vi "LOG Initialize Hardware References.vi"(8 "error in (no error)":errorcluster, 10 "Message Data":variant, 11 "Hardware Resources in":T1) -> (0 "error out":errorcluster, 3 "Hardware Resources out":T1)   [LabVIEW 2020, in "LOG.lvlib"]
doc: "Initialize the hardware references."
uses:
  LOG.lvlib
  LOG Configuration.ctl
  support/Message Queue/Message Cluster.ctl
  support/Message Queue/Message Queue.lvlib
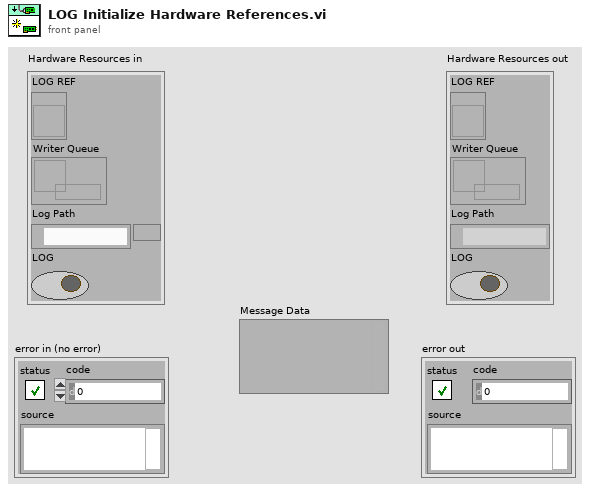
[diagram p1: front panel]
types:
  T1 = typedef "LOG.lvlib/LOG Configuration.ctl" = cluster{"LOG REF":refnum<vi>, "Writer Queue":refnum<queue>, "Log Path":path, "LOG":bool}
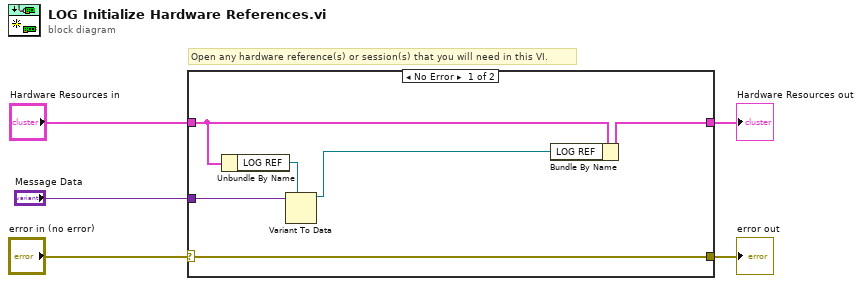
[diagram p0: block diagram]
diagram:
  # "Open any hardware reference(s) or session(s) that you will need in this VI."
  n1 = case shown="No Error" "error in (no error)" {
    selector: "error in (no error)" -> [w6 w12]
    tunnel: [w6 w12] -> w4
    tunnel: "Hardware Resources in" -> [w9 w13]
    tunnel: [w11 w13] -> w2
    tunnel: "Message Data" -> [w10 _]
    frame No Error {
      n2 = Unbundle By Name(w9) -> ("LOG REF"=w8:refnum<vi>)
      n3 = Variant To Data(type=w8, Variant=w10) -> (data=w7:refnum<vi>)  [unwired: 1 in, 1 out]
      n4 = Bundle By Name(cluster=w9, "LOG REF"=w7) -> (w11:T1)
    }
    frame Error {
    }
  }
  "Hardware Resources out" <- w2
  "error out" <- w4
